vi "Select server and param.vi"(0 "Activate":bool) -> (3 "This VI":refnum<vi>, 4 "host out":T1, 6 "HOST OK":bool, 8 "AI table out":string="EP_XQ.1801" caption="таблица аналоговых параметров", 10 "AI":string[](array[string]), 12 "DI OK":bool, 13 "DI":string[](array[string]), 14 "DI table out":string="EP_XQ.1801" caption="таблица дискретных параметров", 15 "AI OK":bool)   [LabVIEW 2019]
uses:
  Database/PostgreSQL2LabVIEW/libpqlv/src/PQconnectdb.vi
  Database/PostgreSQL2LabVIEW/libpqlv/src/PQerrorMessage.vi
  Database/PostgreSQL2LabVIEW/libpqlv/src/PQstatus.vi
  Database/PostgreSQL2LabVIEW/libpqUtility/src/PQgetColumn.vi
  Database/select_initial.vi
  Database/PostgreSQL2LabVIEW/libpqUtility/src/PQclose.vi
  Database/PostgreSQL2LabVIEW/libpqlv/src/PQgetResult.vi
  Database/PostgreSQL2LabVIEW/libpqlv/src/PQclear.vi
  Database/PostgreSQL2LabVIEW/libpqUtility/src/PQfetchTables.vi
  Database/PostgreSQL2LabVIEW/libpqlv/src/PQresultErrorMessage.vi
  Database/PostgreSQL2LabVIEW/libpqlv/src/PQresultStatus.vi
  Database/PostgreSQL2LabVIEW/libpqlv/src/PQsendQuery.vi
  Database/PostgreSQL2LabVIEW/libpqlv/src/PQgetvalue.vi
  Database/PostgreSQL2LabVIEW/libpqlv/src/PQntuples.vi
  Database/PostgreSQL2LabVIEW/libpqUtility/src/PQgetTable.vi
  Database/Progress.vi
  Database/PostgreSQL2LabVIEW/libpqUtility/libpqutility.lvlib
  Database/PostgreSQL2LabVIEW/libpqlv/libpqlv.lvlib
  Inputs.lvlib
panel:
  in  "dbname":string="e101c" caption="база данных"
  in  "AI5":u16(ring)
  in  "AI6":u16(ring)
  in  "AI7":u16(ring)
  in  "AI8":u16(ring)
  in  "AI1":u16(ring)=63
  in  "AI2":u16(ring)=44
  in  "AI3":u16(ring)
  in  "AI4":u16(ring)
  in  "AI9":u16(ring)
  in  "AI10":u16(ring)
  in  "AI6_ON":bool
  in  "AI5_ON":bool
  in  "AI1_ON":bool=TRUE
  in  "AI2_ON":bool=TRUE
  in  "AI3_ON":bool
  in  "AI4_ON":bool
  in  "AI7_ON":bool
  in  "AI8_ON":bool
  in  "AI9_ON":bool
  in  "AI10_ON":bool
  in  "DI10_ON":bool
  in  "DI9_ON":bool
  in  "DI8_ON":bool
  in  "DI7_ON":bool
  in  "DI6_ON":bool
  in  "DI5_ON":bool
  in  "DI4_ON":bool
  in  "DI3_ON":bool
  in  "DI2_ON":bool
  in  "DI1_ON":bool=TRUE
  in  "DI10":u16(ring) items=["GM1FZ1_XB19 "]
  in  "DI9":u16(ring) items=["GM1FZ1_XB19 "]
  in  "DI8":u16(ring) items=["GM1FZ1_XB19 "]
  in  "DI7":u16(ring) items=["GM1FZ1_XB19 "]
  in  "DI6":u16(ring) items=["GM1FZ1_XB19 "]
  in  "DI5":u16(ring) items=["GM1FZ1_XB19 "]
  in  "DI4":u16(ring) items=["GM1FZ1_XB19 "]
  in  "DI3":u16(ring) items=["GM1FZ1_XB19 "]
  in  "DI2":u16(ring) items=["GM1FZ1_XB19 "]
  in  "DI1":u16(ring) items=["GM1FZ1_XB19 "]
  in  "DI0":u16(ring) items=["GM1FZ1_XB19"]
  in  "AI0":u16(ring) items=["GM1QN10_XQ01", "GM1QN11_XQ01", "GM1QN12_XQ01", "GM1QN13_XQ01", "GM1QN14_XQ01", "GM1QN15_XQ01", "GM1QN16_XQ01", "GM1QN17_XQ01", "GM1QN18_XQ01", "GM1QN19_XQ01", "GM1QN1_XQ01", "GM1QN20_XQ01", "GM1QN21_XQ01", "GM1QN22_XQ01", "GM1QN23_XQ01", "GM1QN2_XQ01", "GM1QN3_XQ01", "GM1QN4_XQ01", "GM1QN5_XQ01", "GM1QN6_XQ01", "GM1QN7_XQ01", "GM1QN8_XQ01", "GM1QN9_XQ01"]
  in  "OK":bool
  in  "DI OK curr":bool
  in  "AI OK curr":bool
  in  "HOST OK curr":bool
  out "status":string="нет соединения" caption="состояние"
  in  "connect":bool
  in  "DI table":string="GM1_XB" caption="таблица дискретных параметров"
  in  "AI table":string="AZ1_XQ" caption="таблица аналоговых параметров"
  in  "host":string="localhost" caption="сервер"
  in  "password":string="Pht3833449525" caption="пароль"
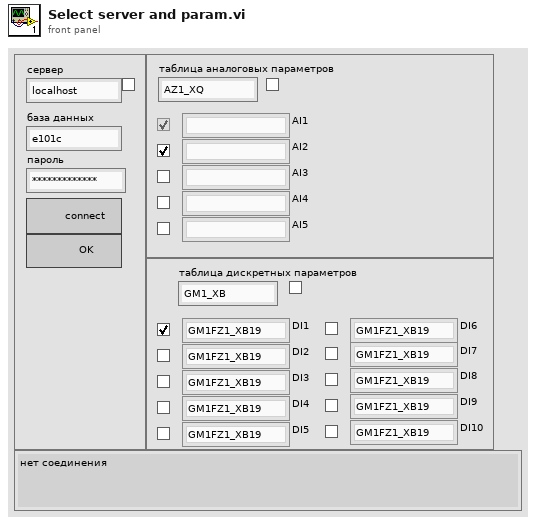
[diagram p1: front panel]
types:
  T1 = cluster{"host":string, "port":string, "client_encoding":string, "dbname":string, "user":string, "password":string}
  T2 = enum32{"Invalid", "Standard", "Closed", "Hidden", "Minimized", "Maximized"}
  T3 = enum32{"CONNECTION_OK", "CONNECTION_BAD", "CONNECTION_STARTED", "CONNECTION_MADE", "CONNECTION_AWAITING_RESPONSE", "CONNECTION_AUTH_OK", "CONNECTION_SETENV", "CONNECTION_SSL_STARTUP", "CONNECTION_NEEDED"}
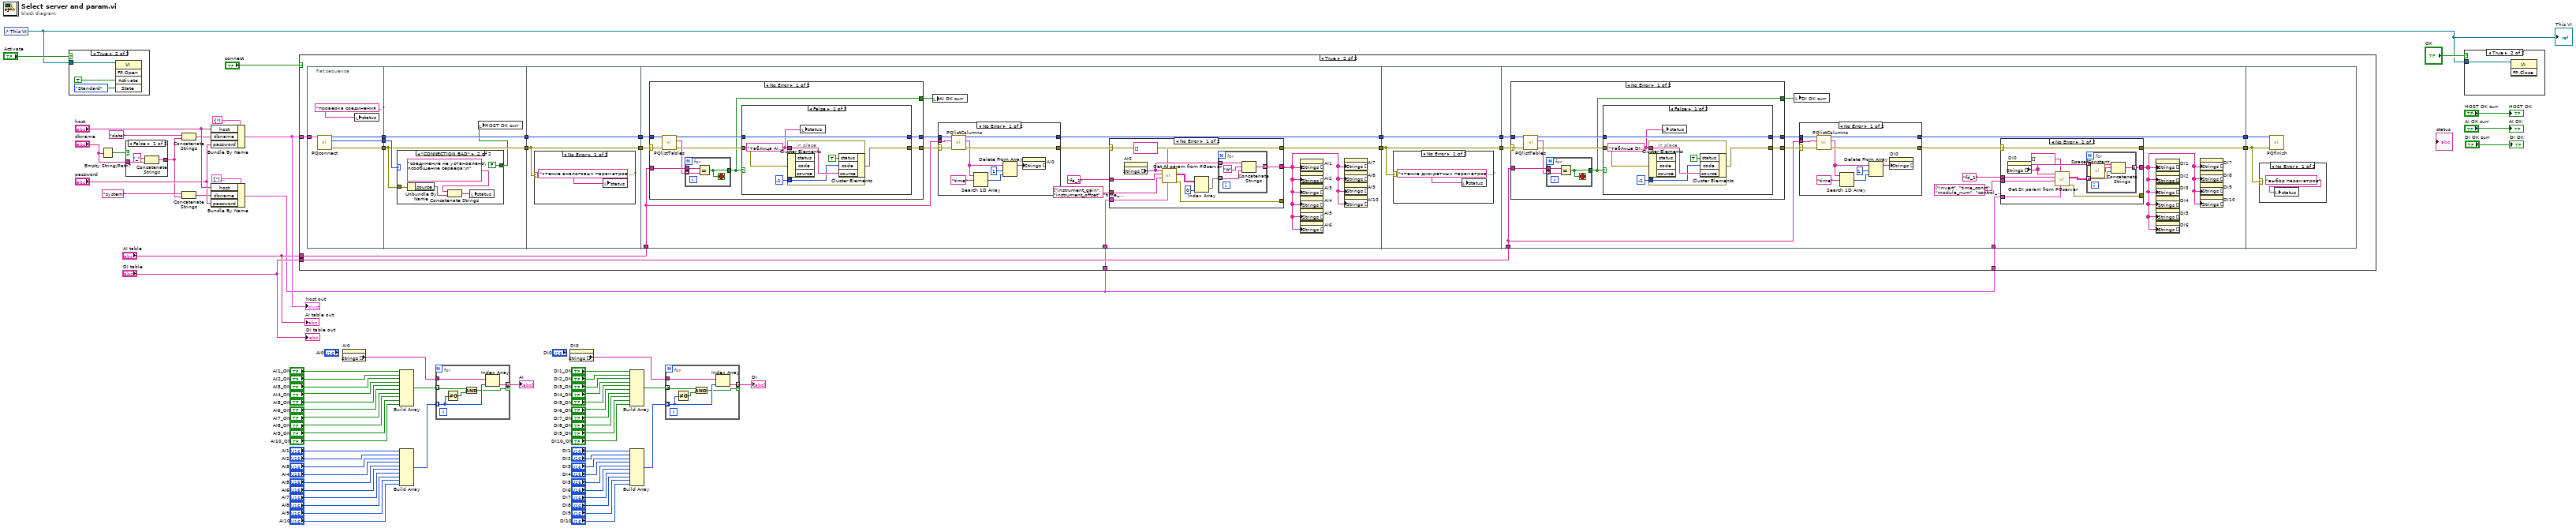
[diagram p0: block diagram]
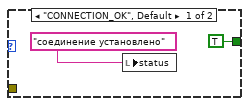
[diagram p4: hidden frame]
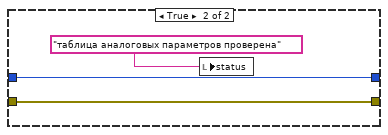
[diagram p8: hidden frame]
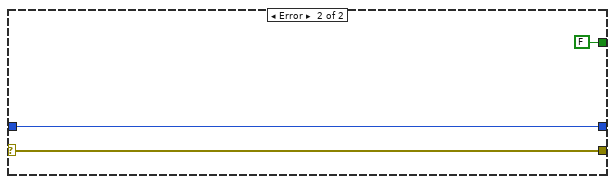
[diagram p9: hidden frame]
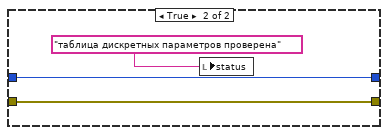
[diagram p13: hidden frame]
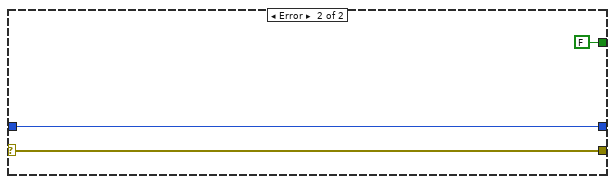
[diagram p14: hidden frame]
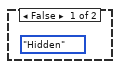
[diagram p16: hidden frame]
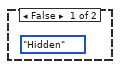
[diagram p17: hidden frame]
diagram:
  n1 = control-ref of="This VI"() -> (w1:refnum<vi>)
  "This VI" <- w1
  n2 = case shown="True" "Activate" {
    tunnel: w1 -> [_ w72]
    frame False {
      (unwired) T2."Hidden" ("State")
    }
    frame True {
      n3 = invoke class="VI" method="FP.Open"(reference=w72, "Activate"=TRUE ("Activate?"), "State"=T2."Standard") -> ()  [unwired: 2 in, 5 out]
    }
  }
  n4 = Empty String/Path?(string/path="dbname") -> (empty?=w10:bool)
  n5 = case shown="False" w10 {
    tunnel: "dbname" -> [w76 w77]
    tunnel: [w74 w77] -> w8
    frame False {
      n6 = Concatenate Strings("_" ("string"), w76) -> (w74:string)
    }
    frame True {
    }
  }
  n7 = Concatenate Strings("data" ("string"), w8) -> (w13:string)
  n8 = Concatenate Strings("system" ("string"), w8) -> (w11:string)
  n9 = Bundle By Name(cluster=T1 {"host"="localhost", "port"="5432", "client_encoding"="LATIN1", "dbname"="data", "user"="postgres", "password"="ghjvfdnj1115"} ("conninfo"), "host"="host", "dbname"=w13, "password"="password") -> (w66:T1)
  "host out" <- w66
  n10 = Bundle By Name(cluster=T1 {"host"="localhost", "port"="5432", "client_encoding"="LATIN1", "dbname"="system", "user"="postgres", "password"="ghjvfdnj1115"} ("conninfo"), "host"="host", "dbname"=w11, "password"="password") -> (w59:T1)
  n11 = case shown="True" "connect" {
    tunnel: w66 -> [_ w84]
    tunnel: "AI table" -> [_ w83]
    tunnel: "DI table" -> [_ w82]
    tunnel: w59 -> [_ w78]
    tunnel: w59 -> [_ w79]
    frame False {
    }
    frame True {
      n12 = flat-sequence {
        tunnel: w84 -> [w98]
        tunnel: [w100] -> w95
        tunnel: [w99] -> w94
        tunnel: [w97] -> w93
        tunnel: w95 -> [w104]
        tunnel: w94 -> [w102]
        tunnel: w93 -> [w103]
        tunnel: [w104] -> w92
        tunnel: [w102] -> w91
        tunnel: w92 -> [w113]
        tunnel: [w113] -> w90
        tunnel: w91 -> [w112]
        tunnel: [w112] -> w89
        tunnel: w90 -> [w127]
        tunnel: w89 -> [w126]
        tunnel: w83 -> [w118]
        tunnel: [w122] -> w88
        tunnel: [w116] -> w87
        tunnel: w79 -> [w121]
        tunnel: w88 -> [w182]
        tunnel: w87 -> [w183]
        tunnel: [w183] -> w86
        tunnel: [w182] -> w85
        tunnel: w86 -> [w197]
        tunnel: w85 -> [w196]
        tunnel: w82 -> [w188]
        tunnel: [w186] -> w81
        tunnel: [w192] -> w80
        tunnel: w78 -> [w191]
        tunnel: w81 -> [w251]
        tunnel: w80 -> [w250]
        frame #0 {
          n13 = call "PQconnect.vi"("conninfo"=w98) -> ("error out"=w99:errorcluster, "PQStatus"=w97:T3, "conn"=w100:u32)  [unwired: 8 in]
          n14 = local write "status"("проверка соединения ..." ("status")) -> ()
        }
        frame #1 {
          n15 = case shown="\"CONNECTION_BAD\"" w103 {
            tunnel: w102 -> [_ w111]
            tunnel: [TRUE FALSE] -> w101
            frame "CONNECTION_OK", Default {
              n16 = local write "status"("соединение установлено" ("status")) -> ()
            }
            frame "CONNECTION_BAD" {
              n17 = Unbundle By Name(w111) -> ("source"=w110:string)
              n18 = Concatenate Strings("соединение не установлено\nсообщение сервера:\n" ("status"), w110) -> (w108:string)
              n19 = local write "status"(w108) -> ()
            }
          }
          n20 = local write "HOST OK curr"(w101) -> ()
        }
        frame #2 {
          n21 = case shown="No Error" w112 {
            frame No Error {
              n22 = local write "status"("чтение аналоговых параметров ..." ("status")) -> ()
            }
            frame Error {
            }
          }
        }
        frame #3 {
          n23 = case shown="No Error" w126 {
            selector: w126 -> [w160 w181]
            tunnel: w127 -> [w161 w180]
            tunnel: [w164 w180] -> w119
            tunnel: [w163 w181] -> w117
            tunnel: w118 -> [w162 _]
            tunnel: [w156 FALSE] -> w125
            frame No Error {
              n24 = call "PQlistTables.vi"("error in"=w160, "conn"=w161) -> ("error out"=w157:errorcluster, "Data"=w159:string[], "conn_out"=w158:u32)  [unwired: 7 in]
              n25 = for {
                tunnel: w159 -> [w166] mode=indexing
                tunnel: w162 -> [w167]
                tunnel: [w165] -> w156
                stop <- w165 stop-if-true
                n26 = Equal?(x=w167, y=w166) -> (x = y?=w165:bool)
              }
              n27 = case shown="False" w156 {
                tunnel: w158 -> [w169 w178]
                tunnel: [w169 w178] -> w164
                tunnel: w157 -> [w170 w177]
                tunnel: [w171 w177] -> w163
                frame False {
                  w168 = "таблица AI отсутствует" ("source")
                  n28 = in-place {
                    in-place-border: w168 -> [w175]
                    in-place-border: -1 ("code") -> [w173]
                    n29 = in-place-cluster #1(w170) -> ()  [unwired: 3 out]
                    n30 = in-place-cluster #1("status"=TRUE, "code"=w173, "source"=w175) -> (w171:errorcluster)
                  }
                  n31 = local write "status"(w168) -> ()
                }
                frame True {
                  n32 = local write "status"("таблица аналоговых параметров проверена" ("status")) -> ()
                }
              }
            }
            frame Error {
            }
          }
          n33 = local write "AI OK curr"(w125) -> ()
          n34 = case shown="No Error" w117 {
            selector: w117 -> [w135 w139]
            tunnel: [w133 w139] -> w115
            tunnel: [w136 w138] -> w116
            tunnel: w119 -> [w137 w138]
            tunnel: w118 -> [w134 _]
            frame No Error {
              n35 = call "PQlistColumns.vi"("error in"=w135, "table"=w134, "conn"=w137) -> ("error out"=w133:errorcluster, "Data"=w131:string[], "conn_out"=w136:u32)  [unwired: 6 in]
              n36 = Search 1D Array(1D array=w131, element="time") -> (index of element=w129:i32)  [unwired: 1 in]
              n37 = Delete From Array(array=w131, length=1, index=w129) -> (array with subset deleted=w128:string[])  [unwired: 1 out]
              n38 = property on="AI0" class="Ring (strict)"("Strings []"=w128) -> ()  [unwired: 2 in, 2 out]
            }
            frame Error {
            }
          }
          n39 = case shown="No Error" w115 {
            selector: w115 -> [w141 w155]
            tunnel: [w148 _] -> _
            tunnel: "fa_1" ("AIParamTable") -> [w150 _]
            tunnel: string[] ["instrument_gain", "instrument_offset", "time_const", "instrument_min_offset", "instrument_range_min", "process_range_min", "process_low_acd", "process_low_alr", "process_high_alr", "process_high_acd", "process_range_max", "instrument_range_max", "instrument_max_offset", "d", "input_register_min", "input_register_max", "input_pv_min", "input_pv_max", "module_num", "control_channel_num", "fname", "process_units"] ("AIParamColumns") -> [w149 _]
            tunnel: w121 -> [w147 _]
            tunnel: [w141 w155] -> w122
            tunnel: [w142 _] -> w120
            frame No Error {
              n40 = property on="AI0" class="Ring (strict)"() -> ("Strings []"=w143:string[])  [unwired: 2 in, 2 out]
              n41 = call "Get AI param from PGserver.vi"("conninfo"=w147, "KFM"=string[] [], "AIParamColumns"=w149, "AIParamTable"=w150, "AIParameters"=w143) -> ("error out"=w148:errorcluster, "Names table"=w145:string[][])  [unwired: 4 in, 1 out]
              n42 = Index Array(array=w145, index (col)=0 ("disabled index (col)")) -> (element=w144:string[])  [unwired: 1 in]
              n43 = for {
                tunnel: w143 -> [w154] mode=indexing
                tunnel: w144 -> [w153] mode=indexing
                tunnel: [w152] -> w142 mode=indexing
                n44 = Concatenate Strings(w154, "\t", w153) -> (w152:string)
              }
            }
            frame Error {
            }
          }
          n45 = property on="AI1" class="Ring (strict)"("Strings []"=w120) -> ()  [unwired: 2 in, 2 out]
          n46 = property on="AI2" class="Ring (strict)"("Strings []"=w120) -> ()  [unwired: 2 in, 2 out]
          n47 = property on="AI3" class="Ring (strict)"("Strings []"=w120) -> ()  [unwired: 2 in, 2 out]
          n48 = property on="AI4" class="Ring (strict)"("Strings []"=w120) -> ()  [unwired: 2 in, 2 out]
          n49 = property on="AI5" class="Ring (strict)"("Strings []"=w120) -> ()  [unwired: 2 in, 2 out]
          n50 = property on="AI6" class="Ring (strict)"("Strings []"=w120) -> ()  [unwired: 2 in, 2 out]
          n51 = property on="AI7" class="Ring (strict)"("Strings []"=w120) -> ()  [unwired: 2 in, 2 out]
          n52 = property on="AI8" class="Ring (strict)"("Strings []"=w120) -> ()  [unwired: 2 in, 2 out]
          n53 = property on="AI9" class="Ring (strict)"("Strings []"=w120) -> ()  [unwired: 2 in, 2 out]
          n54 = property on="AI10" class="Ring (strict)"("Strings []"=w120) -> ()  [unwired: 2 in, 2 out]
        }
        frame #4 {
          n55 = case shown="No Error" w182 {
            frame No Error {
              n56 = local write "status"("чтение дискретных параметров ..." ("status")) -> ()
            }
            frame Error {
            }
          }
        }
        frame #5 {
          n57 = case shown="No Error" w196 {
            selector: w196 -> [w228 w249]
            tunnel: w197 -> [w229 w248]
            tunnel: [w232 w248] -> w189
            tunnel: [w231 w249] -> w187
            tunnel: w188 -> [w230 _]
            tunnel: [w224 FALSE] -> w195
            frame No Error {
              n58 = call "PQlistTables.vi"("error in"=w228, "conn"=w229) -> ("error out"=w225:errorcluster, "Data"=w227:string[], "conn_out"=w226:u32)  [unwired: 7 in]
              n59 = for {
                tunnel: w227 -> [w234] mode=indexing
                tunnel: w230 -> [w235]
                tunnel: [w233] -> w224
                stop <- w233 stop-if-true
                n60 = Equal?(x=w235, y=w234) -> (x = y?=w233:bool)
              }
              n61 = case shown="False" w224 {
                tunnel: w226 -> [w237 w246]
                tunnel: [w237 w246] -> w232
                tunnel: w225 -> [w238 w245]
                tunnel: [w239 w245] -> w231
                frame False {
                  w236 = "таблица DI отсутствует" ("source")
                  n62 = in-place {
                    in-place-border: w236 -> [w243]
                    in-place-border: -1 ("code") -> [w241]
                    n63 = in-place-cluster #2(w238) -> ()  [unwired: 3 out]
                    n64 = in-place-cluster #2("status"=TRUE, "code"=w241, "source"=w243) -> (w239:errorcluster)
                  }
                  n65 = local write "status"(w236) -> ()
                }
                frame True {
                  n66 = local write "status"("таблица дискретных параметров проверена" ("status")) -> ()
                }
              }
            }
            frame Error {
            }
          }
          n67 = local write "DI OK curr"(w195) -> ()
          n68 = case shown="No Error" w187 {
            selector: w187 -> [w205 w209]
            tunnel: [w203 w209] -> w185
            tunnel: [w206 w208] -> w186
            tunnel: w189 -> [w207 w208]
            tunnel: w188 -> [w204 _]
            frame No Error {
              n69 = call "PQlistColumns.vi"("error in"=w205, "table"=w204, "conn"=w207) -> ("error out"=w203:errorcluster, "Data"=w201:string[], "conn_out"=w206:u32)  [unwired: 6 in]
              n70 = Search 1D Array(1D array=w201, element="time") -> (index of element=w199:i32)  [unwired: 1 in]
              n71 = Delete From Array(array=w201, length=1, index=w199) -> (array with subset deleted=w198:string[])  [unwired: 1 out]
              n72 = property on="DI0" class="Ring (strict)"("Strings []"=w198) -> ()  [unwired: 2 in, 2 out]
            }
            frame Error {
            }
          }
          n73 = case shown="No Error" w185 {
            selector: w185 -> [w211 w223]
            tunnel: w191 -> [w216 _]
            tunnel: [w215 _] -> _
            tunnel: "fd_1" ("DIParamTable") -> [w218 _]
            tunnel: string[] ["invert", "time_const", "module_num", "control_channel_num", "fname"] ("DIParamColumns") -> [w217 _]
            tunnel: [w211 w223] -> w192
            tunnel: [w213 _] -> w190
            frame No Error {
              n74 = property on="DI0" class="Ring (strict)"() -> ("Strings []"=w214:string[])  [unwired: 2 in, 2 out]
              n75 = call "Get DI param from PGserver.vi"("conninfo"=w216, "KFM"=string[] [], "DIParamColumns"=w217, "DIParamTable"=w218, "DI_fcode_full"=w214) -> ("error out"=w215:errorcluster, "Names table"=w212:string[][])  [unwired: 4 in, 1 out]
              n76 = for {
                tunnel: w214 -> [w222] mode=indexing
                tunnel: w212 -> [w220] mode=indexing
                tunnel: [w219] -> w213 mode=indexing
                n77 = call <vilib>:"Space Constant.vi"() -> ("String"=w221:string)
                n78 = Concatenate Strings(w222, w221, w220) -> (w219:string)
              }
            }
            frame Error {
            }
          }
          n79 = property on="DI1" class="Ring (strict)"("Strings []"=w190) -> ()  [unwired: 2 in, 2 out]
          n80 = property on="DI2" class="Ring (strict)"("Strings []"=w190) -> ()  [unwired: 2 in, 2 out]
          n81 = property on="DI3" class="Ring (strict)"("Strings []"=w190) -> ()  [unwired: 2 in, 2 out]
          n82 = property on="DI4" class="Ring (strict)"("Strings []"=w190) -> ()  [unwired: 2 in, 2 out]
          n83 = property on="DI5" class="Ring (strict)"("Strings []"=w190) -> ()  [unwired: 2 in, 2 out]
          n84 = property on="DI6" class="Ring (strict)"("Strings []"=w190) -> ()  [unwired: 2 in, 2 out]
          n85 = property on="DI7" class="Ring (strict)"("Strings []"=w190) -> ()  [unwired: 2 in, 2 out]
          n86 = property on="DI8" class="Ring (strict)"("Strings []"=w190) -> ()  [unwired: 2 in, 2 out]
          n87 = property on="DI9" class="Ring (strict)"("Strings []"=w190) -> ()  [unwired: 2 in, 2 out]
          n88 = property on="DI10" class="Ring (strict)"("Strings []"=w190) -> ()  [unwired: 2 in, 2 out]
        }
        frame #6 {
          n89 = case shown="No Error" w250 {
            frame No Error {
              n90 = local write "status"("выбор параметров" ("status")) -> ()
            }
            frame Error {
            }
          }
          n91 = call "PQfinish.vi"("error in (no error)"=w250, "conn"=w251) -> ()  [unwired: 9 in, 1 out]
        }
      }
    }
  }
  n92 = property on="AI0" class="Ring (strict)"() -> ("Strings []"=w16:string[])  [unwired: 2 in, 2 out]
  n93 = Build Array("AI1_ON", "AI2_ON", "AI3_ON", "AI4_ON", "AI5_ON", "AI6_ON", "AI7_ON", "AI8_ON", "AI9_ON", "AI10_ON") -> (w37:bool[])
  n94 = Build Array("AI1", "AI2", "AI3", "AI4", "AI5", "AI6", "AI7", "AI8", "AI9", "AI10") -> (w38:u16[])
  n95 = for {
    tunnel: w16 -> [w258]
    tunnel: w38 -> [w254] mode=indexing
    tunnel: w37 -> [w255] mode=indexing
    tunnel: [w257] -> w7 mode=indexing if=w253
    n96 = Not Equal To 0?(x=w254) -> (x != 0?=w256:bool)
    n97 = And(x=w255, y=w256) -> (x .and. y?=w253:bool)
    n98 = Index Array(array=w258, index=w254) -> (element=w257:string)
  }
  "AI" <- w7
  n99 = property on="DI0" class="Ring (strict)"() -> ("Strings []"=w6:string[])  [unwired: 2 in, 2 out]
  n100 = Build Array("DI1_ON", "DI2_ON", "DI3_ON", "DI4_ON", "DI5_ON", "DI6_ON", "DI7_ON", "DI8_ON", "DI9_ON", "DI10_ON") -> (w5:bool[])
  n101 = Build Array("DI1", "DI2", "DI3", "DI4", "DI5", "DI6", "DI7", "DI8", "DI9", "DI10") -> (w4:u16[])
  n102 = for {
    tunnel: w6 -> [w264]
    tunnel: w4 -> [w260] mode=indexing
    tunnel: w5 -> [w261] mode=indexing
    tunnel: [w263] -> w3 mode=indexing if=w259
    n103 = Not Equal To 0?(x=w260) -> (x != 0?=w262:bool)
    n104 = And(x=w261, y=w262) -> (x .and. y?=w259:bool)
    n105 = Index Array(array=w264, index=w260) -> (element=w263:string)
  }
  "DI" <- w3
  n106 = case shown="True" "OK" {
    tunnel: w1 -> [_ w265]
    frame False {
      (unwired) T2."Hidden" ("State")
    }
    frame True {
      n107 = invoke class="VI" method="FP.Close"(reference=w265) -> ()  [unwired: 2 in, 3 out]
    }
  }
  "HOST OK" <- "HOST OK curr"
  "AI OK" <- "AI OK curr"
  "DI OK" <- "DI OK curr"
  "AI table out" <- "AI table"
  "DI table out" <- "DI table"
